vi "CR-导丝缺损检测3.vi"(8 "error in (no error)":errorcluster caption="错误输入（无错误）", 11 "名称或相对路径":string="Template Program") -> (0 "error in (no error) 2":errorcluster caption="错误输入（无错误）")   [LabVIEW 2017]
uses:
  Picture/SaveButtom.ctl
  Global System.vi
  <vilib>/Utility/xml.llb/Write to XML File(string).vi
panel:
  in  "获取图像":bool
  in  "ROI获取":bool
  in  "创建模板":bool
  in  "保存图像":bool
  out "添加的路径":path
  in  "刷新":bool
  in  "测试按钮":bool
  in  "保存按钮":bool
  in  "Main":enum32{"主参数", "模板匹配参数 ", "测试效果"}(tab)
  in  "导丝缺损检测3基础参数":T1={"IsNorImage"=TRUE, "Exposure Values"=100289, "ImagePath"=path "C:/Users/hedongpo/Desktop/514-hdp/Alignment Assemble System/Test Picture/B/3.bmp"} caption="参数界面" {"Exposure Values" scale=0.0..200000.0}
  in  "导丝缺损检测3参数":T3={"Rectangle"={"Left"=0, "Top"=0, "Right"=0, "Bottom"=0, "Rotation"=0.0}, "Algorithm "=2, "Parameters"={"Number of Matches Requested"=1, "Minimum Match Score"=800.0, "Angle Ranges"=[{"Start Angle"=-180.0, "End Angle"=180.0}]}, "Advanced Options "=[{"Item"=102, "Value"=10.0}, {"Item"=106, "Value"=300.0}, {"Item"=107, "Value"=0.0}, {"Item"=108, "Value"=6.0}, {"Item"=109, "Value"=1.0}, {"Item"=114, "Value"=25.0}, {"Item"=111, "Value"=20.0}, {"Item"=112, "Value"=10.0}, {"Item"=113, "Value"=20.0}, {"Item"=103, "Value"=1.0}, {"Item"=104, "Value"=20.0}, {"Item"=105, "Value"=0.0}, {"Item"=100, "Value"=5.0}], "模板路径"=path "", "Color Plane "=0} {"Color Plane" items=["Red", "Green", "Blue", "Hue", "Saturation", "Luminance", "Value", "Intensity"]; "Advanced Options"."Item" items=["LD Sampling - Minimum Constrast"=0, "LD Sampling - Enable Subpixel Accuracy"=1, "LD Sampling - Search Strategy"=2, "LD Sampling - Subpixel Iterations"=3, "LD Sampling - Subpixel Tolerance"=4, "LD Sampling - Initial Match List Length"=5, "LD Sampling - Match List Reduction Factor"=6, "LD Sampling - Initial Step Size"=7, "LD Sampling - Intermediate Angular Accuracy"=8, "-"=9, "Pyramid - Max Pyramid Level"=100, "Pyramid - Minimum Contrast"=102, "Pyramid - Enable Subpixel Accuracy"=103, "Pyramid - Subpixel Iterations"=104, "Pyramid - Subpixel Tolerance"=105, "Pyramid - Initial Match List Length"=106, "Pyramid - Match List Reduction Factor"=107, "Pyramid - Intermediate Angular Accuracy"=108, "Pyramid - Process Border Matches"=109, "Pyramid - Min Match Separation Distance"=111, "Pyramid - Min Match Separation Angle"=112, "Pyramid - Max Match Overlap"=113, "Pyramid - Max Cache in MB"=114, "Pyramid - Clear Cache"=115, "-"=116, "Enable Defect Map"=200]; "Algorithm" items=["All", "Low Discrepancy Sampling", "Grayscale Value Pyramid", "Gradients Pyramid"]; "Rectangle"."Rotation" format="%.2f"; "Rectangle"."Left" scale=0.0..1024.0; "Rectangle"."Right" scale=0.0..1024.0}
  out "结果":bool
  out "原始图像":T4(plugin-control)
  out "模板图片":T4(plugin-control)
  out "路径输出":path
  in  "Vision Paramter Save Buttom":T5
  out "system time":string
  in  "取消按钮":bool
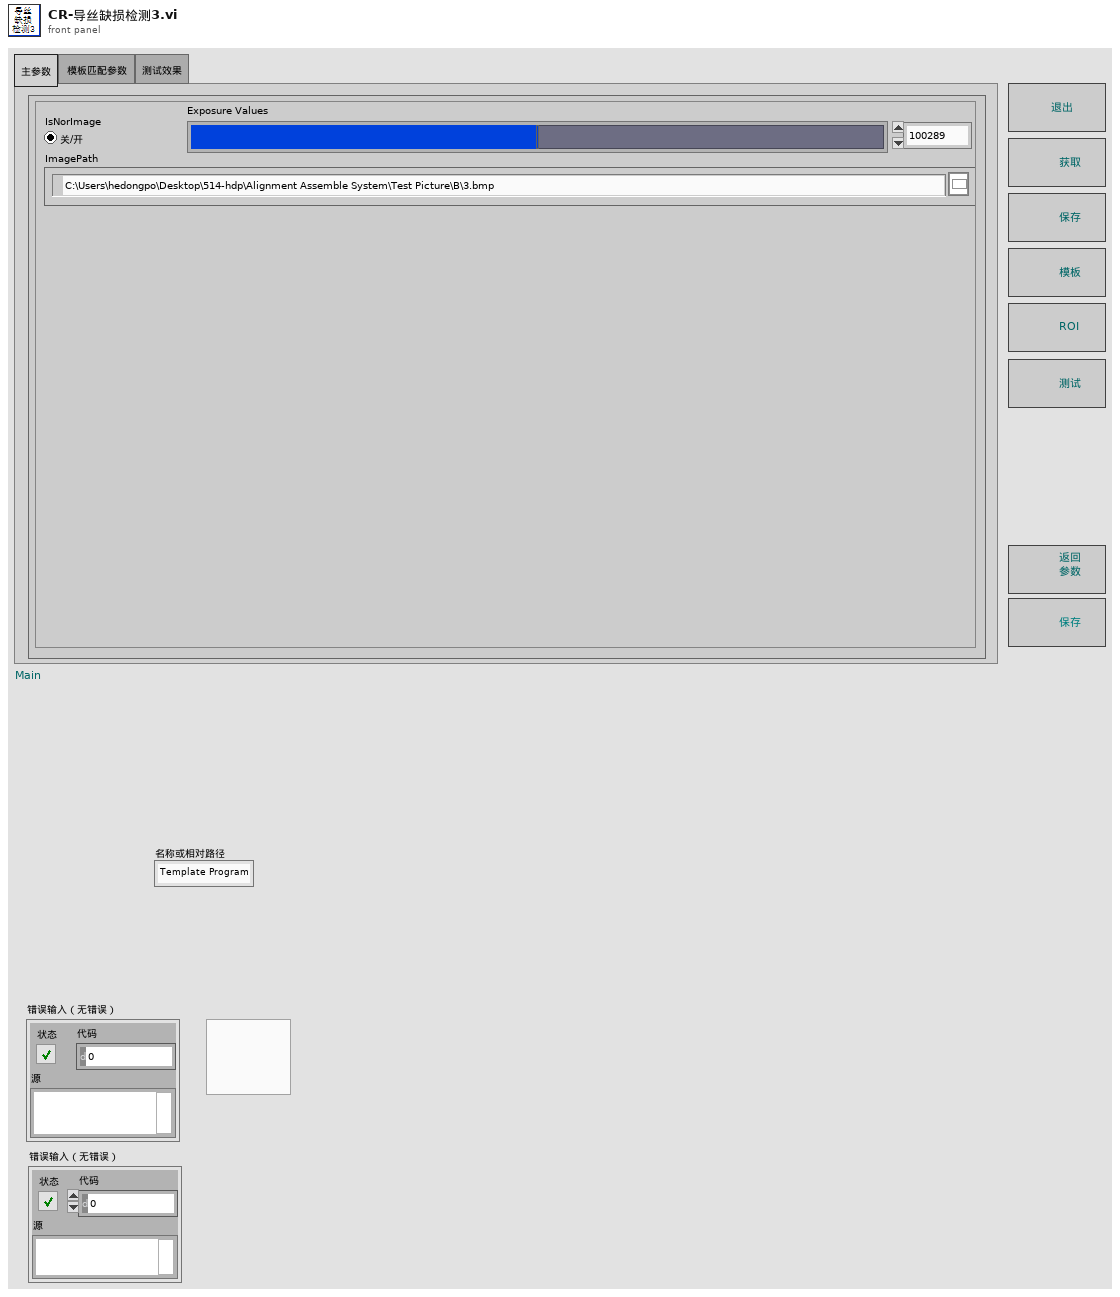
[diagram p1: front panel]
types:
  T1 = cluster{"IsNorImage":bool, "Exposure Values":u32, "ImagePath":path}
  T2 = typedef "IMAQ Rectangle" = cluster{"Left":i32, "Top":i32, "Right":i32, "Bottom":i32, "Rotation":dbl}
  T3 = cluster{"Rectangle":T2, "Algorithm ":i32, "Parameters":cluster{"Number of Matches Requested":i32, "Minimum Match Score":sgl, "Angle Ranges":cluster{"Start Angle":sgl, "End Angle":sgl}[]}, "Advanced Options ":cluster{"Item":u16, "Value":dbl}[], "模板路径":path, "Color Plane ":i32}
  T4 = typedef "IMAQ Image.ctl" = refnum<image>
  T5 = typedef "SaveButtom.ctl" = bool
  T6 = cluster{"index":i32, "this vi":refnum<vi>, "error out":errorcluster}
  T7 = cluster{"master data":string, "priority":u16, "secondary data":string[]}
  T8 = cluster{"case name":string[], "queue array":refnum<queue>[]}
  T9 = typedef "Image Type" = u32
  T10 = cluster{"Global Rectangle":i32[], "Contours":cluster{"Contour Type":u32, "ROI Type":u32, "Points":i32[]}[]}
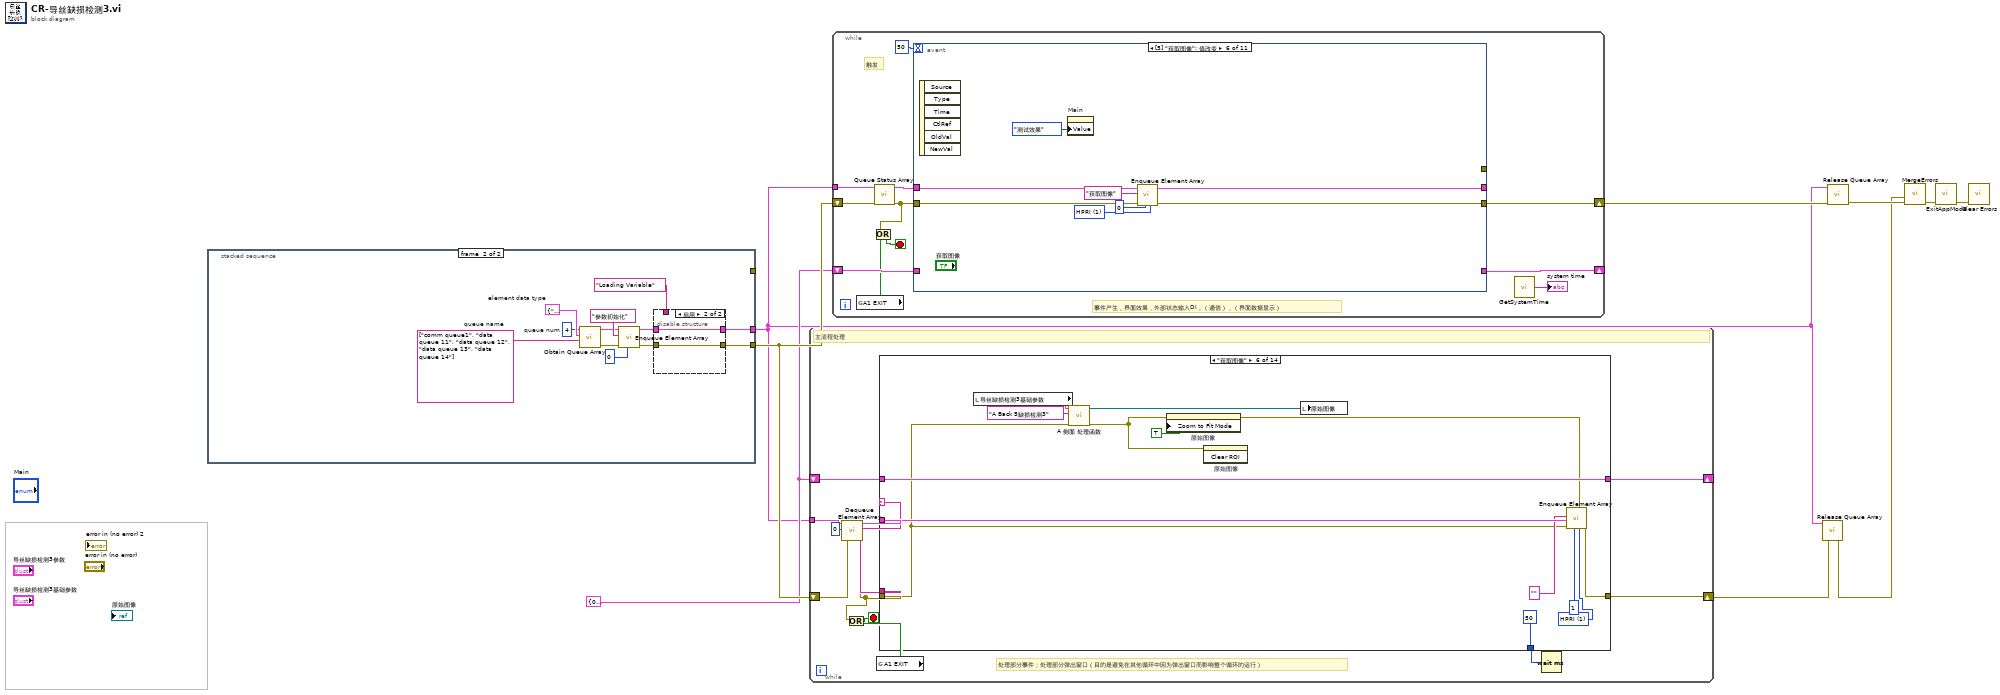
[diagram p0: block diagram]
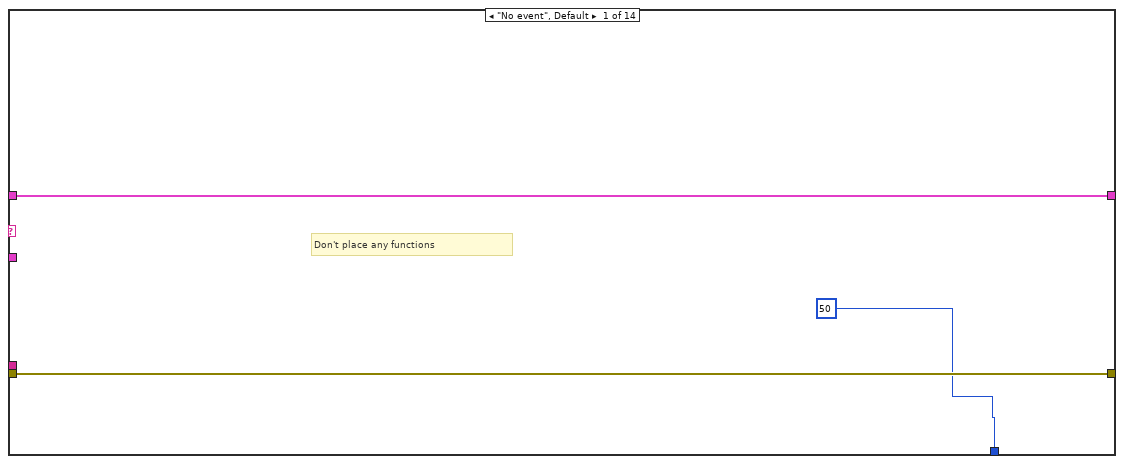
[diagram p2: hidden frame]
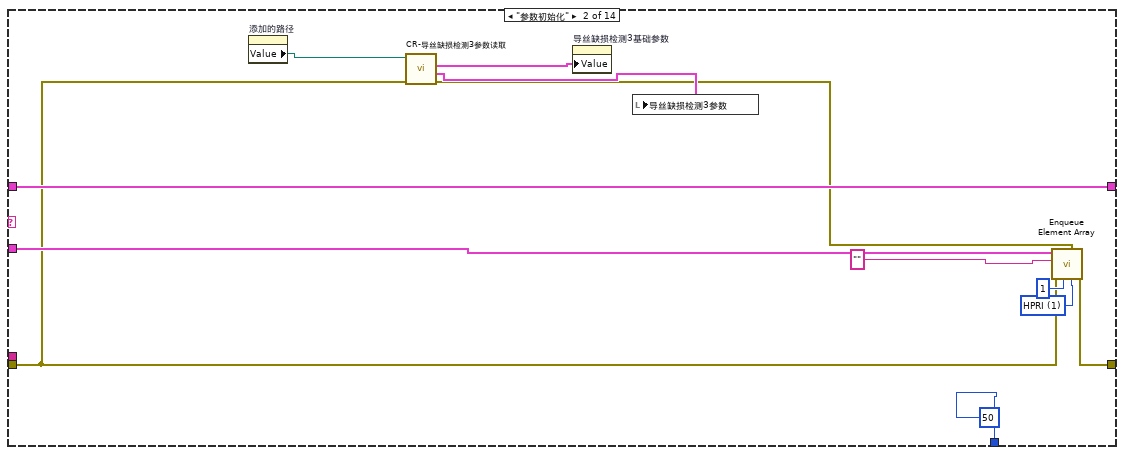
[diagram p3: hidden frame]
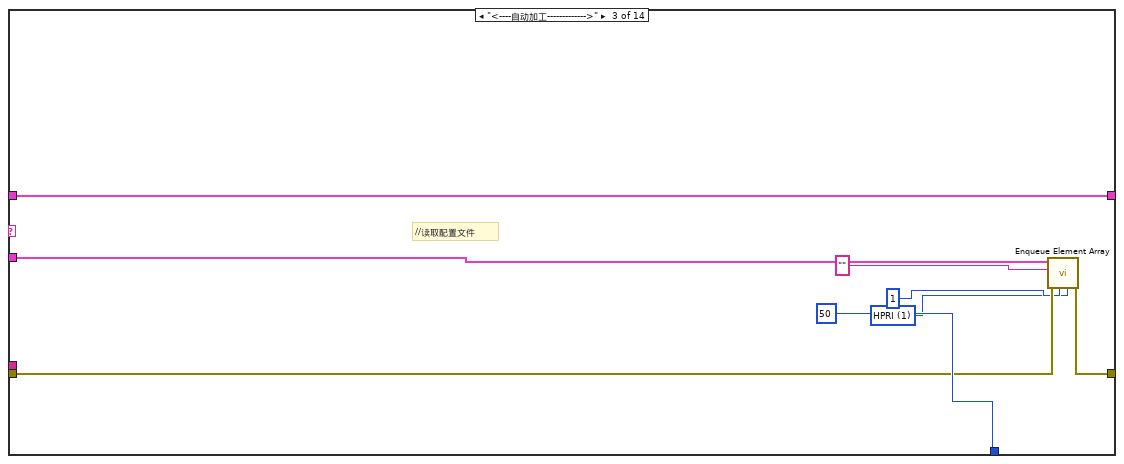
[diagram p4: hidden frame]
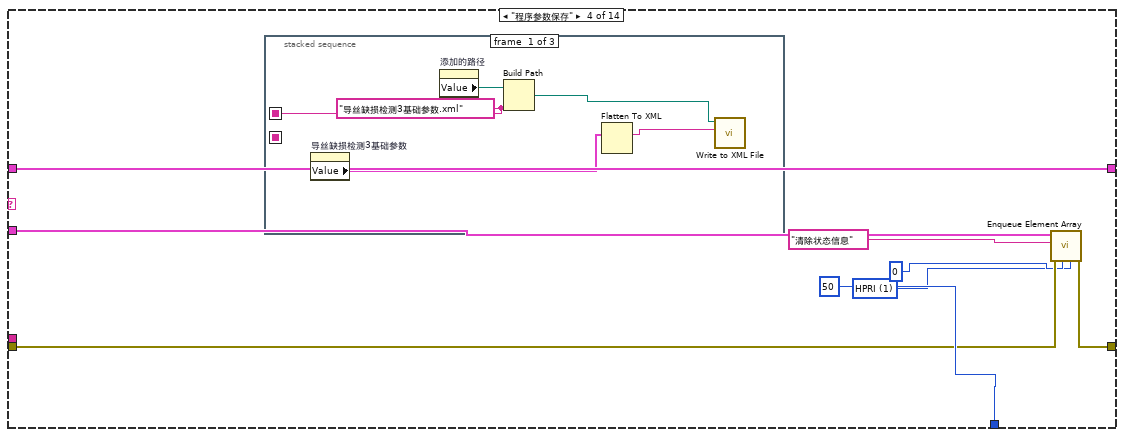
[diagram p5: hidden frame]
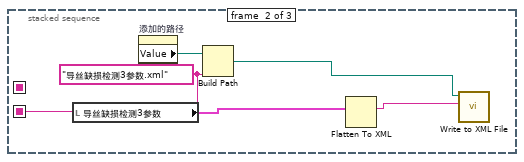
[diagram p6: hidden frame]
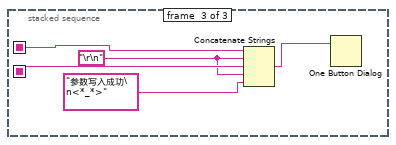
[diagram p7: hidden frame]
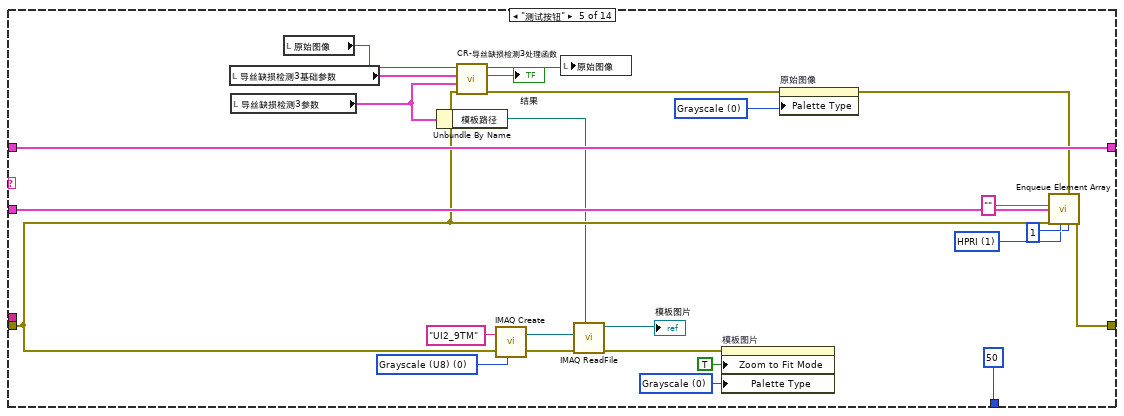
[diagram p8: hidden frame]
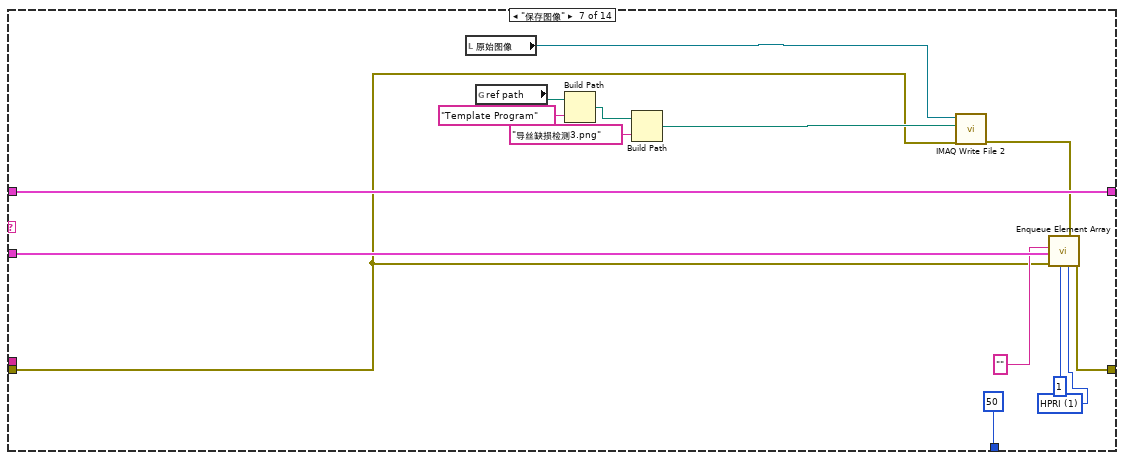
[diagram p9: hidden frame]
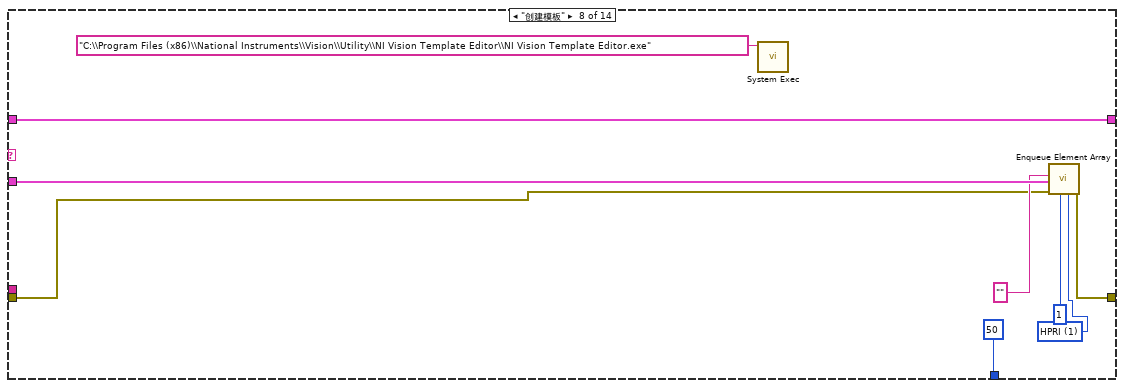
[diagram p10: hidden frame]
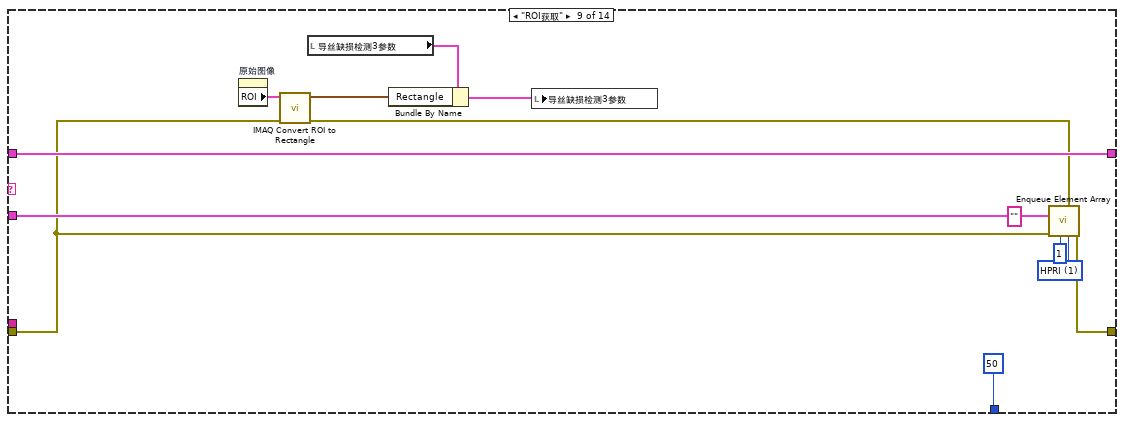
[diagram p11: hidden frame]
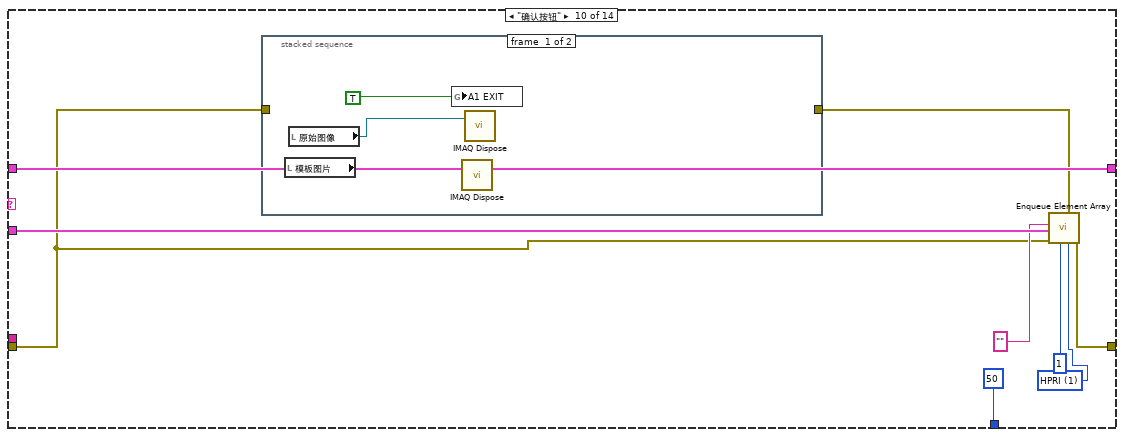
[diagram p12: hidden frame]
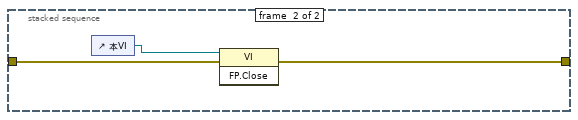
[diagram p13: hidden frame]
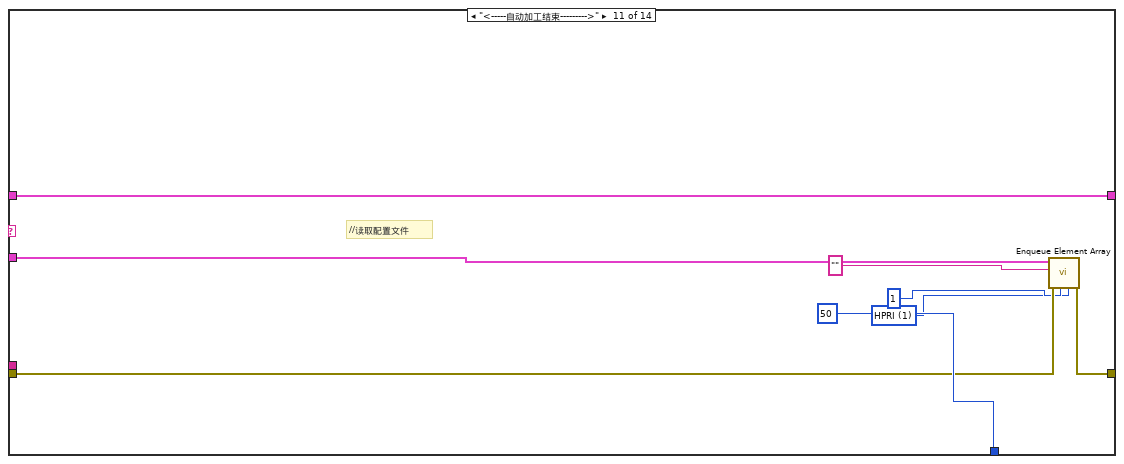
[diagram p14: hidden frame]
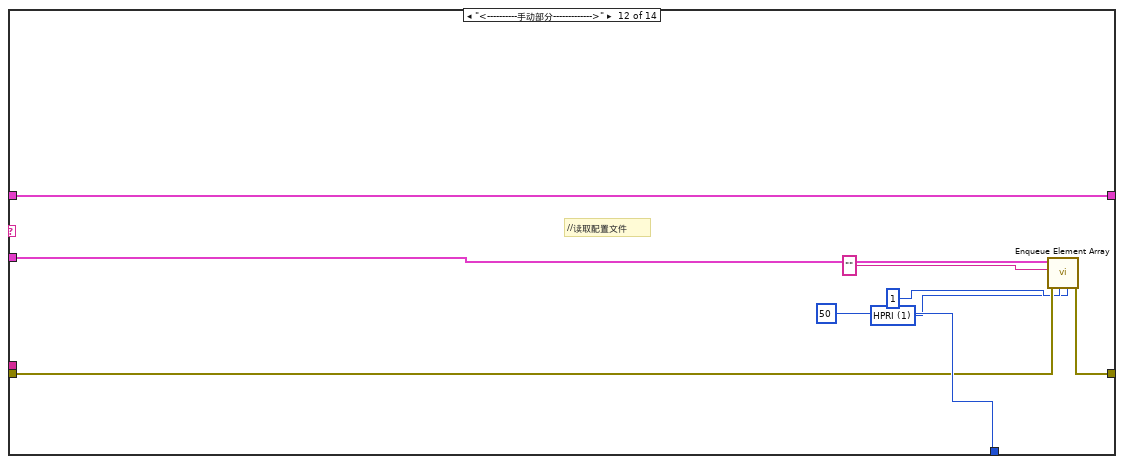
[diagram p15: hidden frame]
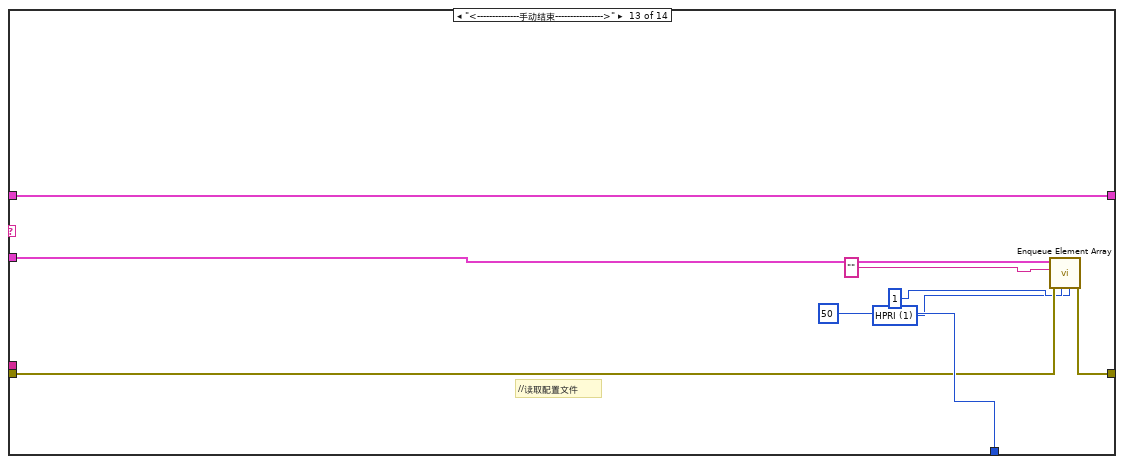
[diagram p16: hidden frame]
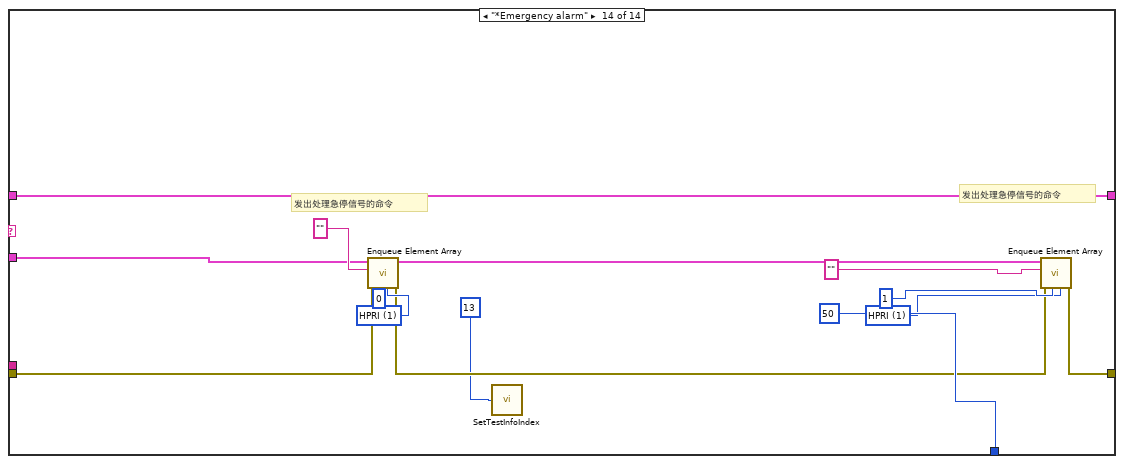
[diagram p17: hidden frame]
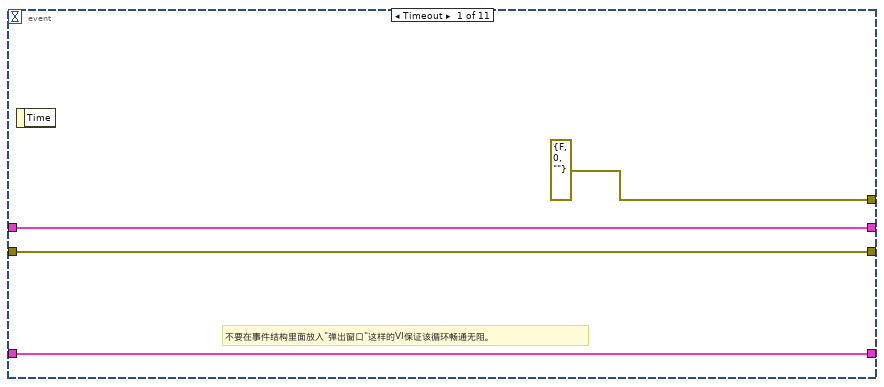
[diagram p18: hidden frame]
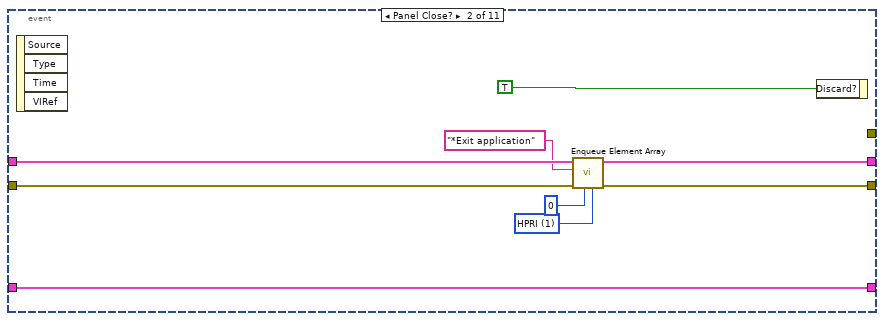
[diagram p19: hidden frame]
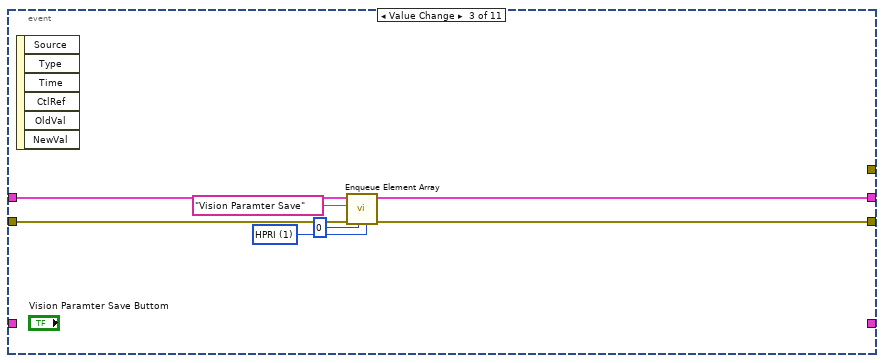
[diagram p20: hidden frame]
diagram:
  w4 = T6 {"index"=0, "this vi"=refnum, "error out"={"status"=FALSE, "code"=0, "source"=""}} ("parameter buffer")
  n1 = stacked-sequence {
    tunnel: [w15 _] -> _
    tunnel: [_ w19] -> w5
    tunnel: [_ w18] -> w1
    frame #0 {
      n2 = global read "Global System.vi" "ref path"() -> (w13:path)
      n3 = Build Path(base path=w13, name or relative path="Template Program" ("名称或相对路径")) -> (appended path=w11:path)
      n4 = property on="Main" class="TabCtl (严格)"("Value"=enum32{"主参数", "模板匹配参数 ", "测试效果"}."主参数" ("Main")) -> ()  [unwired: 2 in, 2 out]
      n5 = Build Path(base path=w11, name or relative path="名称或相对路径") -> (appended path=w17:path)
      "添加的路径" <- w17
      n6 = List Folder(path=w17) -> (path out=→"路径输出":path, error out=w15:errorcluster)  [unwired: 3 in, 2 out]
    }
    frame #1 {
      w27 = string[] ["comm queue1", "data queue 11", "data queue 12", "data queue 13", "data queue 14"]  # queue name
      w28 = 4  # queue num
      w29 = T7 {"master data"="", "priority"=0, "secondary data"=[]}  # element data type
      n7 = call "Obtain Queue Array.vi"("queue name"=w27, "element data type"=w29, "queue num"=w28) -> ("error out"=w23:errorcluster, "queue out"=w24:T8)  [unwired: 2 in, 1 out]
      n8 = call "Enqueue Element Array.vi"("queue index"=0, "error in"=w23, "master data"="参数初始化", "queue in"=w24) -> ("error out"=w22:errorcluster, "queue out"=w21:T8)  [unwired: 6 in]
      n9 = disable-structure shown="启用" {
        disable-tunnel: w22 -> [w35 w36]
        disable-tunnel: w21 -> [w34 w37]
        disable-tunnel: "Loading Variable" ("master data") -> [w33 _]
        disable-tunnel: [w31 w36] -> w19
        disable-tunnel: [w30 w37] -> w18
        frame Disabled {
          n10 = call "Enqueue Element Array.vi"("queue index"=12, "error in"=w35, "master data"=w33, "queue in"=w34) -> ("error out"=w31:errorcluster, "queue out"=w30:T8)  [unwired: 6 in]
        }
        frame Enabled {
        }
      }
    }
  }
  n11 = while {
    shift-right: [w50] -> w3
    shift-left: w5 -> [w41]
    shift-right: [w47] -> _
    shift-left: w4 -> [w48]
    tunnel: w1 -> [w43]
    stop <- w38 stop-if-true
    # "处理部分事件；处理部分弹出窗口（目的是避免在其他循环中因为弹出窗口而影响整个循环的运行）"
    # "主流程处理"
    n12 = call "Dequeue Element Array.vi"("queue in"=w43, "queue index"=0, "error in"=w41) -> ("queue out"=w46:T8, "master data"=w45:string, "secondary data"=w44:string[], "error out"=w40:errorcluster)  [unwired: 2 in, 1 out]
    n13 = global read "Global System.vi" "A1 EXIT"() -> (w39:bool)
    n14 = Or(x=w40, y=w39) -> (x .or. y?=w38:bool)
    n15 = case shown="\"获取图像\"" w45 {
      tunnel: w46 -> [_ w64 w72 w74 w120 w134 w149 w158 w171 w180 w194 w202 w210 w216]
      tunnel: w40 -> [w52 w57 w68 w78 w113 w125 w136 w152 w164 w174 w190 w198 w206 w213]
      tunnel: [w52 w63 w71 w80 w119 w133 w148 w157 w170 w179 w193 w201 w209 w224] -> w50
      tunnel: [50 50 50 50 50 50 50 50 50 50 50 50 50 50] -> w49
      tunnel: w48 -> [w53 w59 w69 w75 w115 w129 w144 w153 w166 w175 w191 w199 w207 w222]
      tunnel: [w53 w59 w69 w75 w115 w129 w144 w153 w166 w175 w191 w199 w207 w222] -> w47
      tunnel: w44 -> [_ _ _ _ _ _ _ _ _ _ _ _ _ _]
      frame "No event", Default {
        # "Don't place any functions"
      }
      frame "参数初始化" {
        w60 = u16 1 items=["HPRI"=1, "LPRI"=0] ("priority")
        n16 = property on="添加的路径" class="Path"() -> ("Value"=w58:path)  [unwired: 2 in, 2 out]
        n17 = call "CR-导丝缺损检测3参数读取.vi"("error in (no error)"=w57, "基路径"=w58) -> ("error out"=w54:errorcluster, "导丝缺损检测3参数"=w55:T3, "导丝缺损检测3基础参数"=w56:T1)  [unwired: 6 in]
        n18 = property on="导丝缺损检测3基础参数" class="Clust (严格)"("Value"=w56) -> ()  [unwired: 2 in, 2 out]
        n19 = local write "导丝缺损检测3参数"(w55) -> ()
        n20 = call "Enqueue Element Array.vi"("priority"=w60, "device error in"=w54, "queue index"=1, "error in"=w57, "master data"="" ("Element 1"), "queue in"=w64) -> ("error out"=w63:errorcluster)  [unwired: 4 in, 1 out]
      }
      frame "<----自动加工------------->" {
        w66 = u16 1 items=["HPRI"=1, "LPRI"=0] ("priority")
        # "//读取配置文件"
        n21 = call "Enqueue Element Array.vi"("priority"=w66, "queue index"=1, "error in"=w68, "master data"="" ("Element 1"), "queue in"=w72) -> ("error out"=w71:errorcluster)  [unwired: 5 in, 1 out]
      }
      frame "程序参数保存" {
        w76 = u16 1 items=["HPRI"=1, "LPRI"=0] ("priority")
        n22 = stacked-sequence {
          seq-local: [w82 _ _] -> [_ _ w95]
          seq-local: [_ w88 _] -> [_ _ w93]
          frame #0 {
            w82 = "导丝缺损检测3基础参数.xml" ("名称或相对路径")
            n23 = property on="导丝缺损检测3基础参数" class="Clust (严格)"() -> ("Value"=w85:T1)  [unwired: 2 in, 2 out]
            n24 = property on="添加的路径" class="Path"() -> ("Value"=w86:path)  [unwired: 2 in, 2 out]
            n25 = Build Path(base path=w86, name or relative path=w82) -> (appended path=w83:path)
            n26 = Flatten To XML(anything=w85) -> (xml string=w84:string)
            n27 = call-poly <vilib>:"Write to XML File.vi"("XML Input"=w84, "XML File Path"=w83) -> ()  [unwired: 7 in, 3 out]
          }
          frame #1 {
            w88 = "导丝缺损检测3参数.xml" ("名称或相对路径")
            n28 = local read "导丝缺损检测3参数"() -> (w87:T3)
            n29 = property on="添加的路径" class="Path"() -> ("Value"=w91:path)  [unwired: 2 in, 2 out]
            n30 = Build Path(base path=w91, name or relative path=w88) -> (appended path=w89:path)
            n31 = Flatten To XML(anything=w87) -> (xml string=w90:string)
            n32 = call-poly <vilib>:"Write to XML File.vi"("XML Input"=w90, "XML File Path"=w89) -> ()  [unwired: 7 in, 3 out]
          }
          frame #2 {
            w92 = "\r\n"
            n33 = Concatenate Strings(w95, w92, w93, w92, "参数写入成功\n<*_*>" ("消息")) -> (w94:string)
            n34 = One Button Dialog(message=w94) -> ()  [unwired: 1 in, 1 out]
          }
        }
        n35 = call "Enqueue Element Array.vi"("priority"=w76, "queue index"=0, "error in"=w78, "master data"="清除状态信息" ("Element 1"), "queue in"=w74) -> ("error out"=w80:errorcluster)  [unwired: 5 in, 1 out]
      }
      frame "测试按钮" {
        w100 = u32 0 items=["Grayscale", "Binary", "Gradient", "Rainbow", "Temperature", "User Defined", "Binary 16 Bit", "Gradient 16 Bit", "Rainbow 16 Bit", "Temperature 16 Bit", "User Defined 16 Bit"] ("Palette:Palette Type")
        w106 = T9 0 items=["Grayscale (U8)", "Grayscale (I16)", "Grayscale (SGL)", "Complex (CSG)", "RGB (U32)", "HSL (U32)", "RGB (U64)", "Grayscale (U16)"] ("Image Type")
        w108 = u32 0 items=["Grayscale", "Binary", "Gradient", "Rainbow", "Temperature", "User Defined", "Binary 16 Bit", "Gradient 16 Bit", "Rainbow 16 Bit", "Temperature 16 Bit", "User Defined 16 Bit"] ("Palette:Palette Type")
        w116 = u16 1 items=["HPRI"=1, "LPRI"=0] ("priority")
        n36 = local read "导丝缺损检测3基础参数"() -> (w114:T1)
        n37 = local read "导丝缺损检测3参数"() -> (w111:T3)
        n38 = local read "原始图像"() -> (w110:T4)
        n39 = Unbundle By Name(w111) -> ("模板路径"=w99:path)
        n40 = call "CR-导丝缺损检测3处理函数.vi"("error in (no error)"=w113, "UI电源线正面标签1参数"=w111, "电源线正面标签1基础参数"=w114, "Image in"=w110) -> ("error out"=w109:errorcluster, "j结果"=→"结果":bool, "Image out"=w112:T4)  [unwired: 4 in, 1 out]
        n41 = call "IMAQ Create"("Image Name"="UI2_9TM", "Image Type"=w106, "error in (no error)"=w113) -> ("New Image"=w105:T4, "error out"=w104:errorcluster)  [unwired: 2 in]
        n42 = local write "原始图像"(w112) -> ()
        n43 = call "IMAQ ReadFile"("File Path"=w99, "error in (no error)"=w104, "Image"=w105) -> ("error out"=w102:errorcluster, "Image Out"=→"模板图片":T4)  [unwired: 4 in, 3 out]
        n44 = property on="模板图片" class="ImageControl"(error in=w102, "Zoom to Fit Mode"=TRUE, "Palette Type"=w100) -> ()  [unwired: 1 in, 2 out]
        n45 = property on="原始图像" class="ImageControl"(error in=w109, "Palette Type"=w108) -> (error out=w97:errorcluster)  [unwired: 1 in, 1 out]
        n46 = call "Enqueue Element Array.vi"("priority"=w116, "device error in"=w97, "queue index"=1, "error in"=w113, "master data"="" ("Element 1"), "queue in"=w120) -> ("error out"=w119:errorcluster)  [unwired: 4 in, 1 out]
      }
      frame "获取图像" {
        w130 = u16 1 items=["HPRI"=1, "LPRI"=0] ("priority")
        n47 = local read "导丝缺损检测3基础参数"() -> (w127:T1)
        n48 = call "A 侧面 处理函数.vi"("error in (no error)"=w125, "Image Name"="A Back 5缺损检测3", "ParamsUI"=w127) -> ("error out"=w122:errorcluster, "Image out"=w126:T4)  [unwired: 5 in, 2 out]
        n49 = property on="原始图像" class="ImageControl"(error in=w122, "Zoom to Fit Mode"=TRUE) -> (error out=w123:errorcluster)  [unwired: 1 in, 1 out]
        n50 = invoke on="原始图像" class="ImageControl" method="Clear ROI"(error in=w122) -> ()  [unwired: 2 in, 3 out]
        n51 = local write "原始图像"(w126) -> ()
        n52 = call "Enqueue Element Array.vi"("priority"=w130, "device error in"=w123, "queue index"=1, "error in"=w125, "master data"="" ("Element 1"), "queue in"=w134) -> ("error out"=w133:errorcluster)  [unwired: 4 in, 1 out]
      }
      frame "保存图像" {
        w145 = u16 1 items=["HPRI"=1, "LPRI"=0] ("priority")
        n53 = local read "原始图像"() -> (w137:T4)
        n54 = global read "Global System.vi" "ref path"() -> (w143:path)
        n55 = Build Path(base path=w143, name or relative path="Template Program" ("名称或相对路径")) -> (appended path=w141:path)
        n56 = Build Path(base path=w141, name or relative path="导丝缺损检测3.png" ("名称或相对路径")) -> (appended path=w139:path)
        n57 = call-poly "IMAQ Write File 2"("error in (no error)"=w136, "File Path"=w139, "Image"=w137) -> ("error out"=w138:errorcluster)  [unwired: 7 in, 1 out]
        n58 = call "Enqueue Element Array.vi"("priority"=w145, "device error in"=w138, "queue index"=1, "error in"=w136, "master data"="" ("Element 1"), "queue in"=w149) -> ("error out"=w148:errorcluster)  [unwired: 4 in, 1 out]
      }
      frame "创建模板" {
        w154 = u16 1 items=["HPRI"=1, "LPRI"=0] ("priority")
        n59 = call <vilib>:"System Exec.vi"("command line"="C:\\Program Files (x86)\\National Instruments\\Vision\\Utility\\NI Vision Template Editor\\NI Vision Template Editor.exe") -> ()  [unwired: 7 in, 4 out]
        n60 = call "Enqueue Element Array.vi"("priority"=w154, "queue index"=1, "error in"=w152, "master data"="" ("Element 1"), "queue in"=w158) -> ("error out"=w157:errorcluster)  [unwired: 5 in, 1 out]
      }
      frame "ROI获取" {
        w167 = u16 1 items=["HPRI"=1, "LPRI"=0] ("priority")
        n61 = property on="原始图像" class="ImageControl"() -> ("ROI"=w165:T10)  [unwired: 2 in, 2 out]
        n62 = call "IMAQ Convert ROI to Rectangle"("error in (no error)"=w164, "ROI Descriptor"=w165) -> ("error out"=w160:errorcluster, "Rectangle"=w162:T2)  [unwired: 7 in]
        n63 = local read "导丝缺损检测3参数"() -> (w163:T3)
        n64 = Bundle By Name(cluster=w163, "Rectangle"=w162) -> (w161:T3)
        n65 = local write "导丝缺损检测3参数"(w161) -> ()
        n66 = call "Enqueue Element Array.vi"("priority"=w167, "device error in"=w160, "queue index"=1, "error in"=w164, "master data"="" ("Element 1"), "queue in"=w171) -> ("error out"=w170:errorcluster)  [unwired: 4 in, 1 out]
      }
      frame "确认按钮" {
        w176 = u16 1 items=["HPRI"=1, "LPRI"=0] ("priority")
        n67 = stacked-sequence {
          tunnel: w174 -> [_ w186]
          tunnel: [_ w185] -> w173
          frame #0 {
            n68 = local read "模板图片"() -> (w182:T4)
            n69 = local read "原始图像"() -> (w183:T4)
            n70 = global write "Global System.vi" "A1 EXIT"(TRUE ("EXIT")) -> ()
            n71 = call "IMAQ Dispose"("Image"=w182) -> ()  [unwired: 5 in, 1 out]
            n72 = call "IMAQ Dispose"("Image"=w183) -> ()  [unwired: 5 in, 1 out]
          }
          frame #1 {
            n73 = control-ref of="本VI"() -> (w187:refnum<vi>)
            n74 = invoke class="VI" method="FP.Close"(reference=w187, error in=w186) -> (error out=w185:errorcluster)  [unwired: 1 in, 2 out]
          }
        }
        n75 = call "Enqueue Element Array.vi"("priority"=w176, "device error in"=w173, "queue index"=1, "error in"=w174, "master data"="" ("Element 1"), "queue in"=w180) -> ("error out"=w179:errorcluster)  [unwired: 4 in, 1 out]
      }
      frame "<-----自动加工结束--------->" {
        w188 = u16 1 items=["HPRI"=1, "LPRI"=0] ("priority")
        # "//读取配置文件"
        n76 = call "Enqueue Element Array.vi"("priority"=w188, "queue index"=1, "error in"=w190, "master data"="" ("Element 1"), "queue in"=w194) -> ("error out"=w193:errorcluster)  [unwired: 5 in, 1 out]
      }
      frame "<----------手动部分------------->" {
        w196 = u16 1 items=["HPRI"=1, "LPRI"=0] ("priority")
        # "//读取配置文件"
        n77 = call "Enqueue Element Array.vi"("priority"=w196, "queue index"=1, "error in"=w198, "master data"="" ("Element 1"), "queue in"=w202) -> ("error out"=w201:errorcluster)  [unwired: 5 in, 1 out]
      }
      frame "<--------------手动结束---------------->" {
        w204 = u16 1 items=["HPRI"=1, "LPRI"=0] ("priority")
        # "//读取配置文件"
        n78 = call "Enqueue Element Array.vi"("priority"=w204, "queue index"=1, "error in"=w206, "master data"="" ("Element 1"), "queue in"=w210) -> ("error out"=w209:errorcluster)  [unwired: 5 in, 1 out]
      }
      frame "*Emergency alarm" {
        w219 = u16 1 items=["HPRI"=1, "LPRI"=0] ("priority")
        w220 = u16 1 items=["HPRI"=1, "LPRI"=0] ("priority")
        # "发出处理急停信号的命令"
        # "发出处理急停信号的命令"
        n79 = call "Enqueue Element Array.vi"("priority"=w219, "queue index"=0, "error in"=w213, "master data"="" ("Element 1"), "queue in"=w216) -> ("error out"=w214:errorcluster, "queue out"=w215:T8)  [unwired: 5 in]
        n80 = call "SetTestInfoIndex.vi"("test info index"=13) -> ()
        n81 = call "Enqueue Element Array.vi"("priority"=w220, "queue index"=1, "error in"=w214, "master data"="" ("Element 1"), "queue in"=w215) -> ("error out"=w224:errorcluster)  [unwired: 5 in, 1 out]
      }
    }
    n82 = Wait (ms)(milliseconds to wait=w49) -> ()  [unwired: 1 out]
  }
  n83 = while {
    shift-right: [w229] -> w6
    shift-left: w5 -> [w233]
    shift-right: [w231] -> _
    shift-left: w4 -> [w232]
    tunnel: w1 -> [w235]
    stop <- w226 stop-if-true
    # "触发"
    # "事件产生，界面效果，外部状态输入DI，（通信），（界面数据显示）"
    n84 = global read "Global System.vi" "A1 EXIT"() -> (w227:bool)
    n85 = call "Queue Status Array.vi"("error in (no error)"=w233, "queue in"=w235) -> ("error out"=w228:errorcluster, "queue out"=w230:T8)  [unwired: 4 in]
    n86 = Or(x=w228, y=w227) -> (x .or. y?=w226:bool)
    n87 = event shown="[5] \"获取图像\": 值改变" {
      selector: _ -> [_ _ _ _ _ _ _ _ _ _ _]
      dyn-events: _ -> [_ _ _ _ _ _ _ _ _ _ _]
      timeout: 50 -> [_ _ _ _ _ _ _ _ _ _ _]
      tunnel: w232 -> [w240 w248 _ _ _ _ _ _ _ _ _]
      tunnel: [w240 w248 _ _ _ _ _ _ _ _ _] -> w231
      tunnel: [errorcluster {"status"=FALSE, "code"=0, "source"=""} ("error out") _ _ _ _ _ _ _ _ _ _] -> _
      tunnel: w230 -> [w238 w247 w253 w260 w267 w275 w282 w289 w297 w305 w313]
      tunnel: w228 -> [w237 w246 w252 w259 w266 w274 w281 w288 w296 w304 w312]
      tunnel: [w237 w245 w250 w257 w264 w272 w279 w286 w294 w302 w310] -> w229
      tunnel: [w238 w244 w251 w258 w265 w273 w280 w287 w295 w303 w311] -> _
      event Timeout {
        # "不要在事件结构里面放入\"弹出窗口\"这样的VI保证该循环畅通无阻。"
        n88 = event-data() -> ()  [unwired: 1 in, 1 out]
      }
      event Panel Close? {
        w242 = u16 1 items=["HPRI"=1, "LPRI"=0] ("priority")
        n89 = event-data() -> ()  [unwired: 1 in, 4 out]
        n90 = call "Enqueue Element Array.vi"("priority"=w242, "queue index"=0, "error in"=w246, "master data"="*Exit application", "queue in"=w247) -> ("error out"=w245:errorcluster, "queue out"=w244:T8)  [unwired: 5 in]
        n91 = event-data("Discard?"=TRUE) -> ()  [unwired: 1 in, 1 out]
      }
      event Value Change {
        w255 = u16 1 items=["HPRI"=1, "LPRI"=0] ("priority")
        n92 = event-data() -> ()  [unwired: 1 in, 6 out]
        n93 = call "Enqueue Element Array.vi"("priority"=w255, "queue index"=0, "error in"=w252, "master data"="Vision Paramter Save", "queue in"=w253) -> ("error out"=w250:errorcluster, "queue out"=w251:T8)  [unwired: 5 in]
      }
      event "取消按钮": Value Change {
        w262 = u16 1 items=["HPRI"=1, "LPRI"=0] ("priority")
        n94 = event-data() -> ()  [unwired: 1 in, 6 out]
        n95 = call "Enqueue Element Array.vi"("priority"=w262, "queue index"=0, "error in"=w259, "master data"="确认按钮", "queue in"=w260) -> ("error out"=w257:errorcluster, "queue out"=w258:T8)  [unwired: 5 in]
      }
      event "保存按钮": Value Change {
        w269 = u16 1 items=["HPRI"=1, "LPRI"=0] ("priority")
        n96 = event-data() -> ()  [unwired: 1 in, 6 out]
        n97 = call "Enqueue Element Array.vi"("priority"=w269, "queue index"=0, "error in"=w266, "master data"="程序参数保存", "queue in"=w267) -> ("error out"=w264:errorcluster, "queue out"=w265:T8)  [unwired: 5 in]
      }
      event "获取图像": Value Change {
        w277 = u16 1 items=["HPRI"=1, "LPRI"=0] ("priority")
        n98 = event-data() -> ()  [unwired: 1 in, 6 out]
        n99 = property on="Main" class="TabCtl (严格)"("Value"=enum32{"主参数", "模板匹配参数 ", "测试效果"}."测试效果" ("Main")) -> ()  [unwired: 2 in, 2 out]
        n100 = call "Enqueue Element Array.vi"("priority"=w277, "queue index"=0, "error in"=w274, "master data"="获取图像", "queue in"=w275) -> ("error out"=w272:errorcluster, "queue out"=w273:T8)  [unwired: 5 in]
      }
      event "保存图像": Value Change {
        w284 = u16 1 items=["HPRI"=1, "LPRI"=0] ("priority")
        n101 = event-data() -> ()  [unwired: 1 in, 6 out]
        n102 = call "Enqueue Element Array.vi"("priority"=w284, "queue index"=0, "error in"=w281, "master data"="保存图像", "queue in"=w282) -> ("error out"=w279:errorcluster, "queue out"=w280:T8)  [unwired: 5 in]
      }
      event "创建模板": Value Change {
        w291 = u16 1 items=["HPRI"=1, "LPRI"=0] ("priority")
        n103 = event-data() -> ()  [unwired: 1 in, 6 out]
        n104 = call "Enqueue Element Array.vi"("priority"=w291, "queue index"=0, "error in"=w288, "master data"="创建模板", "queue in"=w289) -> ("error out"=w286:errorcluster, "queue out"=w287:T8)  [unwired: 5 in]
      }
      event "ROI获取": Value Change {
        w299 = u16 1 items=["HPRI"=1, "LPRI"=0] ("priority")
        n105 = event-data() -> ()  [unwired: 1 in, 6 out]
        n106 = property on="Main" class="TabCtl (严格)"("Value"=enum32{"主参数", "模板匹配参数 ", "测试效果"}."模板匹配参数 " ("Main")) -> ()  [unwired: 2 in, 2 out]
        n107 = call "Enqueue Element Array.vi"("priority"=w299, "queue index"=0, "error in"=w296, "master data"="ROI获取", "queue in"=w297) -> ("error out"=w294:errorcluster, "queue out"=w295:T8)  [unwired: 5 in]
      }
      event "测试按钮": Value Change {
        w307 = u16 1 items=["HPRI"=1, "LPRI"=0] ("priority")
        n108 = event-data() -> ()  [unwired: 1 in, 6 out]
        n109 = property on="Main" class="TabCtl (严格)"("Value"=enum32{"主参数", "模板匹配参数 ", "测试效果"}."测试效果" ("Main")) -> ()  [unwired: 2 in, 2 out]
        n110 = call "Enqueue Element Array.vi"("priority"=w307, "queue index"=0, "error in"=w304, "master data"="测试按钮", "queue in"=w305) -> ("error out"=w302:errorcluster, "queue out"=w303:T8)  [unwired: 5 in]
      }
      event "刷新": Value Change {
        n111 = event-data() -> ()  [unwired: 1 in, 6 out]
        n112 = disable-structure shown="禁用" {
          disable-tunnel: w313 -> [w317 _]
          disable-tunnel: w312 -> [w316 _]
          disable-tunnel: [w315 _] -> w311
          disable-tunnel: [w314 _] -> w310
          frame Disabled {
            w319 = u16 1 items=["HPRI"=1, "LPRI"=0] ("priority")
            # "刷新"
            n113 = call "Enqueue Element Array.vi"("priority"=w319, "queue index"=0, "error in"=w316, "master data"="刷新", "queue in"=w317) -> ("error out"=w314:errorcluster, "queue out"=w315:T8)  [unwired: 5 in]
          }
          frame Enabled {
          }
        }
        n114 = property on="Main" class="TabCtl (严格)"("Value"=enum32{"主参数", "模板匹配参数 ", "测试效果"}."模板匹配参数 " ("Main")) -> ()  [unwired: 2 in, 2 out]
      }
    }
    n115 = call "GetSystemTime.vi"() -> ("date/time string"=→"system time":string)  [unwired: 7 in]
  }
  n116 = call "Release Queue Array.vi"("error in"=w3, "queue in"=w1) -> ("error out"=w2:errorcluster)  [unwired: 2 in, 3 out]
  n117 = call "Release Queue Array.vi"("error in"=w6, "queue in"=w1) -> ("error out"=w9:errorcluster)  [unwired: 2 in, 3 out]
  n118 = call "MergeErrors.vi"("error in 3 (no error)"=w2, "error in 4 (no error)"=w9) -> ("error out"=w8:errorcluster)  [unwired: 6 in]
  n119 = call "ExitAppMode.vi"("error in (no error)"=w8) -> ("error out"=w7:errorcluster)  [unwired: 10 in]
  n120 = call <vilib>:"Clear Errors.vi"("error in (no error)"=w7) -> ()  [unwired: 5 in, 2 out]
